vi "Autosize Tree Get All.vi"(7 "Tree Ref":refnum<vi>, 9 "Number of Columns":i32=31, 11 "error in (no error)":errorcluster) -> (8 "Tree Ref out":refnum<vi>, 10 "Tree Data":string[][](array[string]), 15 "error out":errorcluster)   [LabVIEW 2015]
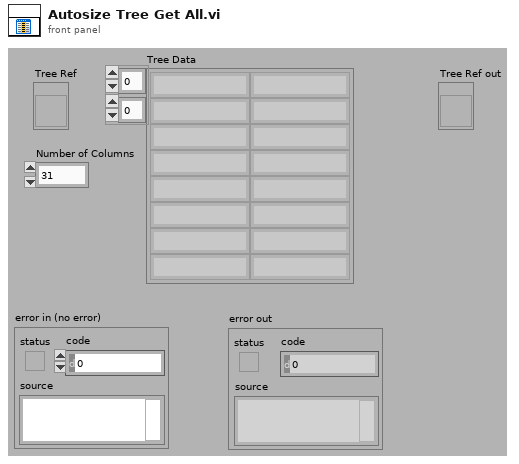
[diagram p1: front panel]
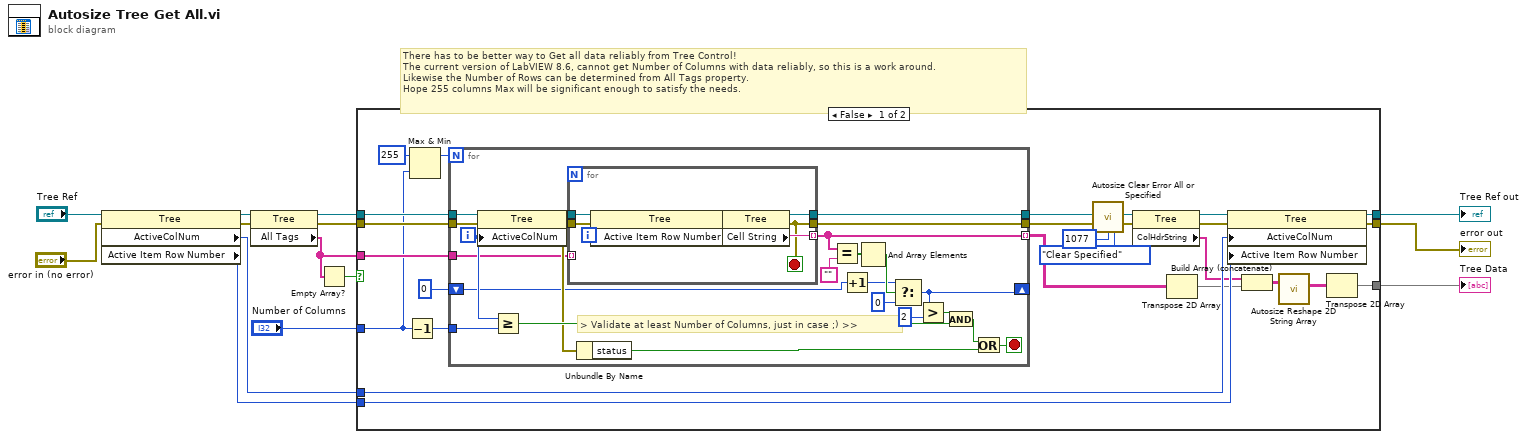
[diagram p0: block diagram]
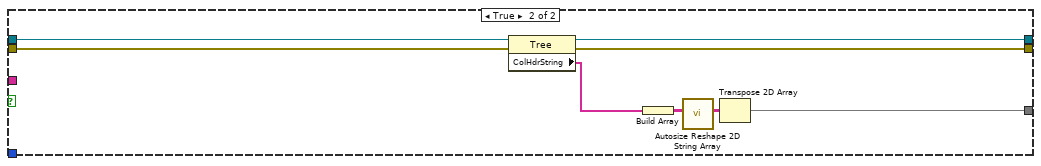
[diagram p2: hidden frame]
diagram:
  # "There has to be better way to Get all data reliably from Tree Control!\nThe current version of LabVIEW 8.6, cannot get Number of Columns with data reliably, so this is a work around. \nLikewise the Number of Rows can be determined from All Tags property.\nHope 255 columns Max will be significant enough to satisfy the needs."
  n1 = property class="Tree"(reference="Tree Ref", error in="error in (no error)") -> (reference out=w8:refnum<vi>, error out=w7:errorcluster, "ActiveColNum"=w6:i32, "Active Item Row Number"=w5:i32)
  n2 = property class="Tree"(reference=w8, error in=w7) -> (reference out=w14:refnum<vi>, error out=w13:errorcluster, "All Tags"=w1:string[])
  n3 = Empty Array?(array=w1) -> (empty?=w4:bool)
  n4 = case shown="False" w4 {
    tunnel: w14 -> [w39 w77]
    tunnel: w13 -> [w38 w78]
    tunnel: [w37 w76] -> w12
    tunnel: [w36 w75] -> w11
    tunnel: w6 -> [w35 _]
    tunnel: w5 -> [w34 _]
    tunnel: [w21 w71] -> w3
    tunnel: "Number of Columns" -> [w16 _]
    tunnel: w1 -> [w18 _]
    frame False {
      n5 = Decrement(x=w16) -> (x-1=w20:i32)
      n6 = Max & Min(x=255, y=w16) -> (max(x,y)=w15:i32)  [unwired: 1 out]
      n7 = for {
        N: w15 -> [_]
        tunnel: [w57] -> w25 mode=indexing
        tunnel: w39 -> [w59]
        tunnel: w38 -> [w60]
        tunnel: [w62] -> w30
        tunnel: [w61] -> w33
        tunnel: w20 -> [w49]
        shift-right: [w42] -> _
        shift-left: 0 -> [w46]
        tunnel: w18 -> [w40]
        i -> [w55]
        stop <- w50 stop-if-true
        # "> Validate at least Number of Columns, just in case ;) >>"
        n8 = property class="Tree"(reference=w59, error in=w60, "ActiveColNum"=w55) -> (reference out=w58:refnum<vi>, error out=w52:errorcluster)
        n9 = Greater Or Equal?(x=w55, y=w49) -> (x >= y?=w53:bool)
        n10 = for {
          tunnel: [w65] -> w57 mode=indexing
          tunnel: w58 -> [w69]
          tunnel: w52 -> [w68]
          tunnel: [w64] -> w62
          tunnel: [w63] -> w61
          tunnel: w40 -> [_] mode=indexing
          i -> [w70]
          stop <- w63 stop-if-true
          n11 = property class="Tree"(reference=w69, error in=w68, "Active Item Row Number"=w70) -> (reference out=w67:refnum<vi>, error out=w66:errorcluster)
          n12 = property class="Tree"(reference=w67, error in=w66) -> (reference out=w64:refnum<vi>, error out=w63:errorcluster, "Cell String"=w65:string)
        }
        n13 = Unbundle By Name(w52) -> ("status"=w51:bool)
        n14 = Equal?(x=w57, y="") -> (x = y?=w54:bool[])
        n15 = Increment(x=w46) -> (x+1=w45:i32)
        n16 = And Array Elements(Boolean array=w54) -> (logical AND=w47:bool)
        n17 = Select(t=w45, s=w47, f=0) -> (s? t:f=w42:i32)
        n18 = Greater?(x=w42, y=2) -> (0:w43:bool)
        n19 = And(x=w43, y=w53) -> (x .and. y?=w48:bool)
        n20 = Or(x=w48, y=w51) -> (x .or. y?=w50:bool)
      }
      n21 = call "Autosize Clear Error All or Specified.vi"("Clear Mode (0: Clear All)"=enum16{"Clear All", "Clear Specified"}."Clear Specified", "Code to Clear (0)"=1077, "error in (no error)"=w33) -> ("error out"=w29:errorcluster)  [unwired: 1 in, 11 out]
      n22 = property class="Tree"(reference=w30, error in=w29) -> (reference out=w28:refnum<vi>, error out=w27:errorcluster, "ColHdrString"=w26:string[])
      n23 = Transpose 2D Array(2D array=w25) -> (transposed array=w24:string[][])
      n24 = property class="Tree"(reference=w28, error in=w27, "ActiveColNum"=w35, "Active Item Row Number"=w34) -> (reference out=w37:refnum<vi>, error out=w36:errorcluster)
      n25 = Build Array (concatenate)(w26, w24) -> (w23:string[][])
      n26 = call "Autosize Reshape 2D String Array.vi"("Array in"=w23) -> ("Array out"=w22:string[][])  [unwired: 10 out]
      n27 = Transpose 2D Array(2D array=w22) -> (transposed array=w21:string[][])
    }
    frame True {
      n28 = property class="Tree"(reference=w77, error in=w78) -> (reference out=w76:refnum<vi>, error out=w75:errorcluster, "ColHdrString"=w74:string[])
      n29 = Build Array(w74) -> (w73:string[][])
      n30 = call "Autosize Reshape 2D String Array.vi"("Array in"=w73) -> ("Array out"=w72:string[][])  [unwired: 10 out]
      n31 = Transpose 2D Array(2D array=w72) -> (transposed array=w71:string[][])
    }
  }
  "Tree Data" <- w3
  "error out" <- w11
  "Tree Ref out" <- w12
